vi "generate_input_parametric.vi"() -> (0 "Z Matrix":dbl[][](array[numeric]), 1 "Y Matrix":dbl[][](array[numeric]), 2 "X Matrix":dbl[][](array[numeric]))   [LabVIEW 2020, in "3DPC_SurfacePlot.xctl"]
uses:
  <vilib>/Native 3D Graph/xcontrol/3DPC_SurfacePlot.xctl
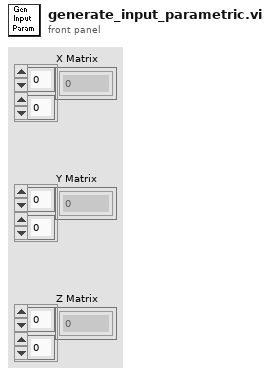
[diagram p1: front panel]
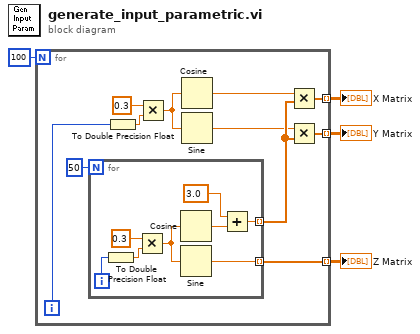
[diagram p0: block diagram]
diagram:
  n1 = for {
    N: 100 -> [_]
    tunnel: [w10] -> w3 mode=indexing
    tunnel: [w9] -> w1 mode=indexing
    tunnel: [w8] -> w2 mode=indexing
    i -> [w5]
    n2 = for {
      N: 50 -> [_]
      tunnel: [w23] -> w14 mode=indexing
      tunnel: [w17] -> w8 mode=indexing
      i -> [w18]
      n3 = To Double Precision Float(number=w18) -> (double precision float=w21:dbl)
      n4 = Multiply(x=0.3, y=w21) -> (x*y=w19:dbl)
      n5 = Cosine(x=w19) -> (cos(x)=w16:dbl)
      n6 = Sine(x=w19) -> (sin(x)=w17:dbl)
      n7 = Add(x=3.0, y=w16) -> (x+y=w23:dbl)
    }
    n8 = To Double Precision Float(number=w5) -> (double precision float=w6:dbl)
    n9 = Multiply(x=0.3, y=w6) -> (x*y=w13:dbl)
    n10 = Cosine(x=w13) -> (cos(x)=w12:dbl)
    n11 = Sine(x=w13) -> (sin(x)=w11:dbl)
    n12 = Multiply(x=w12, y=w14) -> (x*y=w10:dbl[])
    n13 = Multiply(x=w11, y=w14) -> (x*y=w9:dbl[])
  }
  "X Matrix" <- w3
  "Y Matrix" <- w1
  "Z Matrix" <- w2
